vi "_Simulator SWI Tree.vi"   [LabVIEW 2011]
uses:
  SWI Command.ctl
panel:
  # "See Diagram"
types:
  T1 = typedef "SWI Command.ctl" = enum16{"LOAD", "INITIALIZE", "PRESET", "SET STIMULUS", "GET STIMULUS", "GET INFO", "RELEASE", "UNLOAD"}
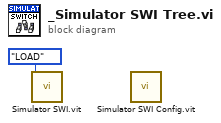
[diagram p0: block diagram]
diagram:
  n1 = call "Simulator SWI.vit"("SWI Command"=SWI_Command."LOAD" ("VNA Command")) -> ()  [unwired: 3 in, 8 out]
  n2 = call "Simulator SWI Config.vit"() -> ()  [unwired: 2 in, 10 out]
